vi "Pulse Fetch Data.vi"(0 "RFmx Session in":refnum<k21>, 11 "error in":errorcluster) -> (3 "Per Pulse Results (Header Name)":string[](array[string]), 4 "RFmx Session Out":refnum<k21>, 6 "Per Pulse Results (for MP)":dbl[][](array[numeric])=[[-60.19434452056885, -48.23559761047363, -61.500163078308105, -61.676697731018066, -50.09932041168213, -61.2670373916626, -47.940940856933594, -60.594682693481445, -54.222588539123535, -68.17487716674805], [-51.47902011871338, -63.676371574401855, -49.32386875152588, -42.60602951049805, -41.78941249847412, -56.57611846923828, -67.04894065856934, -44.43309783935547, -53.89562129974365, -45.59821605682373], [-50.93127727508545, -48.11325550079346, -49.06841278076172, -42.55256652832031, -41.191606521606445, -55.30652046203613, -47.88793087005615, -44.32924270629883, -51.04572772979736, -45.574283599853516], [0.7774313706217917, 0.7743052754564207, 0.6733820768651879, 0.6972024148638998, 0.6739289285829677, 0.8012453172128895, 0.7789831746751243, 0.81331101938709, 0.6993593760935255, 0.7751122603266651], [-0.04818759954671978, -0.17045354969029822, -0.2937592841444876, -0.18006245433349588, -0.30206692305208827, -0.23840372056041464, -0.22733917807886903, -0.2726908323785403, -0.20409866605988866, -0.22706977878895118], [1.8971785430084185, 1.7078184861447125, 1.6125145446758244, 1.6429880662265446, 1.7003339064410368, 1.645767369340552, 1.8225724908268657, 1.500202053052531, 1.816586601520762, 1.7434164608706486], [9.902169056670972e-09, 1.0171003831640633e-08, 1.0087378671871648e-08, 1.0018839745468426e-08, 1.0021453073999283e-08, 9.937162678335199e-09, 1.0113660404718986e-08, 9.936247799288367e-09, 1.0029181489475149e-08, 1.0014254033422958e-08], [1.1747647026741224e-08, 0.00010001147191839247, 0.00020001407632828564, 0.0003000116995963527, 0.00040001415077715896, 0.0005000116894758734, 0.0006000140392077577, 0.000700011761394561, 0.0008000141195439436, 0.000900014054837663], [1.0266075038352937e-08, 1.0210194009332553e-08, 9.96602777140197e-09, 1.0195131948175912e-08, 1.0214687343427613e-08, 1.0248380139892106e-08, 1.003600972591812e-08, 1.0209683835273609e-08, 1.0208458229471944e-08, 1.0051256216333969e-08], [2.0016060941649103e-05, 0.00012001605265167608, 0.0002200186251165217, 0.0003200161244125173, 0.00042001858918951285, 0.0005200161200707459, 0.000620018587380489, 0.0007200160772447398, 0.0008200186061427676, 0.0009200186490169424], [1.9999915173664064e-05, 1.9999928162649538e-05, 1.9999979315091006e-05, 1.9999962883326592e-05, 1.9999940266618827e-05, 1.9999970715330443e-05, 1.9999948164994597e-05, 1.999989449659788e-05, 1.9999961878396942e-05, 2.0000044728873845e-05], [8.000006128542082e-05, 8.000009557087724e-05, 8.000003688745302e-05, 8.000002009960112e-05, 8.000005863752275e-05, 8.000001971001538e-05, 8.000010310677254e-05, 8.000006664992009e-05, 8.000000105017845e-05, nan], [19.999919881828227, 19.999923415962357, 19.999976074586076, 19.99996628673531, 19.99994048578986, 19.999972630258657, 19.999937910673005, 19.999902267256314, 19.99996929267048, nan], [9.999997645908488e-05, 0.00010000002373352679, 0.00010000001620254403, 9.999998298292771e-05, 9.999999890414157e-05, 9.999999042534582e-05, 0.00010000005127176714, 9.999996114651797e-05, 9.99999629285754e-05, nan]], 8 "TS Intrapulse Stability":dbl[][](array[numeric]), 10 "TS P2P Stability":dbl[][](array[numeric]), 14 "TS Acquired Amplitude":dbl[][](array[numeric]), 15 "error out":errorcluster)   [LabVIEW 2023]
uses:
  <vilib>/RFmx/Pulse/mx/RFmxPulse.llb/RFmxPulse Fetch Intrapulse Stability Trace.vi
  <vilib>/RFmx/Pulse/mx/RFmxPulse.llb/RFmxPulse Fetch Pulse To Pulse Stability Trace.vi
  <vilib>/RFmx/Pulse/mx/RFmxPulse.llb/RFmxPulse Fetch Acquired Amplitude Trace.vi
  <resource>/objmgr/RFmxPulse.rc
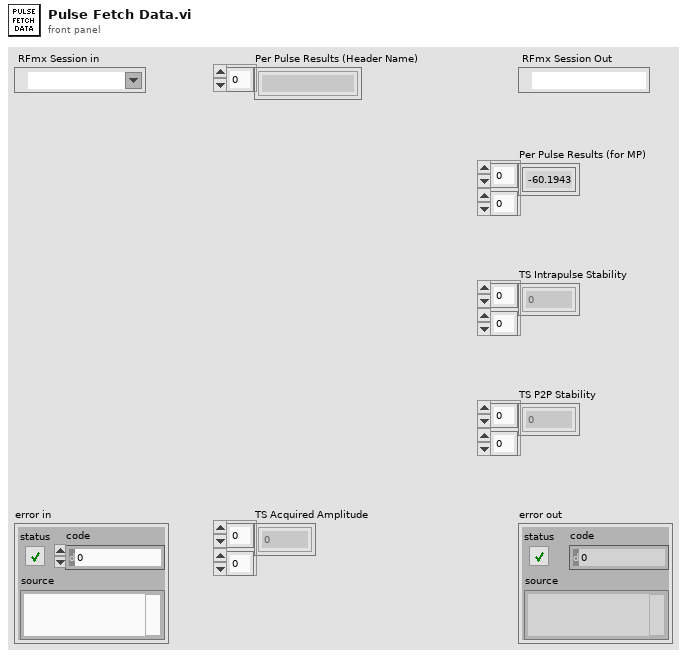
[diagram p1: front panel]
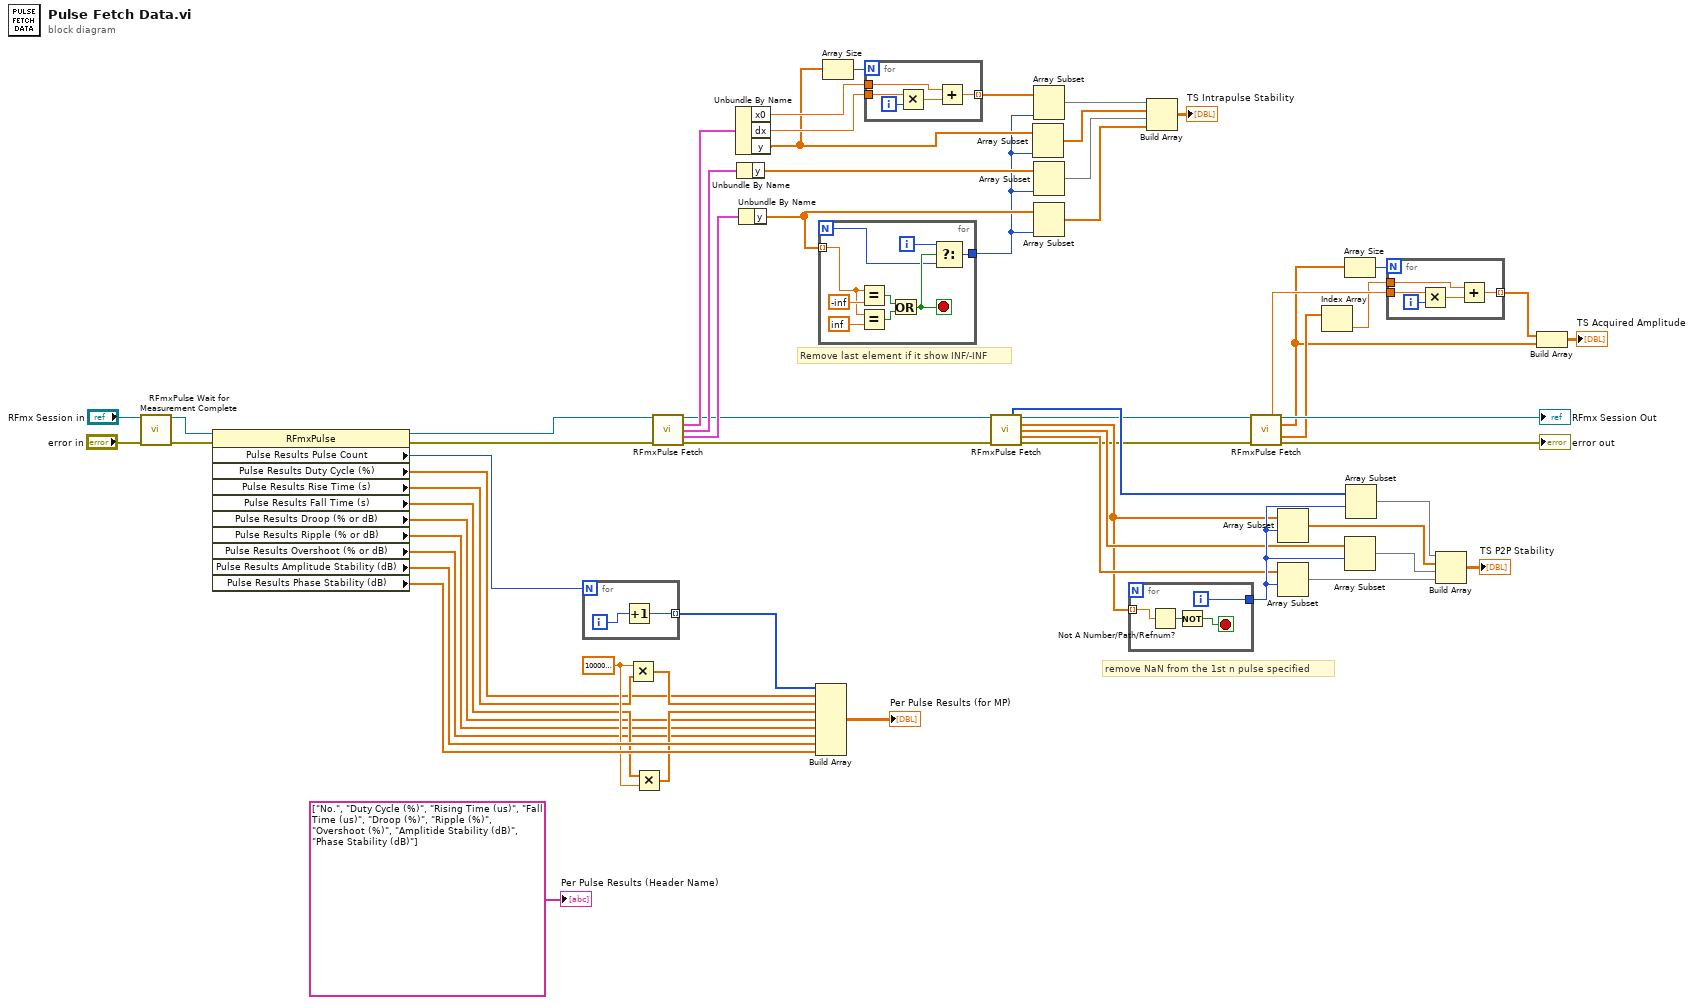
[diagram p0: block diagram]
diagram:
  w30 = 1000000.0
  # "Remove last element if it show INF/-INF"
  # "remove NaN from the 1st n pulse specified"
  n1 = call <vilib>:"RFmxPulse Wait for Measurement Complete.vi"("Instrument Handle In"="RFmx Session in", "error in (no error)"="error in") -> ("Instrument Handle Out"=w17:refnum<k21>, "error out"=w16:errorcluster)  [unwired: 12 in]
  n2 = property class="RFmxPulse"(reference=w17, error in=w16) -> (reference out=w13:refnum<k21>, error out=w14:errorcluster, "Pulse Results Pulse Count"=w37:i32, "Pulse Results Duty Cycle (%)"=w21:dbl[], "Pulse Results Rise Time (s)"=w26:dbl[], "Pulse Results Fall Time (s)"=w28:dbl[], "Pulse Results Droop (% or dB)"=w22:dbl[], "Pulse Results Ripple (% or dB)"=w23:dbl[], "Pulse Results Overshoot (% or dB)"=w24:dbl[], "Pulse Results Amplitude Stability (dB)"=w39:dbl[], "Pulse Results Phase Stability (dB)"=w40:dbl[])
  n3 = for {
    N: w37 -> [_]
    tunnel: [w61] -> w38 mode=indexing
    i -> [w62]
    n4 = Increment(x=w62) -> (x+1=w61:i32)
  }
  n5 = Multiply(x=w30, y=w26) -> (x*y=w27:dbl[])
  n6 = Multiply(x=w28, y=w30) -> (x*y=w29:dbl[])
  n7 = call-poly <vilib>:"RFmxPulse Fetch.vi"("Instrument Handle In"=w13, "error in (no error)"=w14) -> ("Instrument Handle Out"=w18:refnum<k21>, "Intrapulse Amplitude Stability (dB)"=w49:cluster{"x0":dbl, "dx":dbl, "y":sgl[]}, "Intrapulse Phase Stability (dB)"=w47:cluster{"x0":dbl, "dx":dbl, "y":sgl[]}, "Intrapulse Total Stability (dB)"=w45:cluster{"x0":dbl, "dx":dbl, "y":sgl[]}, "error out"=w19:errorcluster)  [unwired: 9 in]
  n8 = Unbundle By Name(w49) -> ("x0"=w53:dbl, "dx"=w52:dbl, "y"=w51:sgl[])
  n9 = Unbundle By Name(w47) -> ("y"=w48:sgl[])
  n10 = Unbundle By Name(w45) -> ("y"=w46:sgl[])
  n11 = Build Array(w38, w21, w27, w29, w22, w23, w24, w39, w40) -> (→"Per Pulse Results (for MP)":dbl[][])
  n12 = for {
    N -> [w63]
    tunnel: w46 -> [w70] mode=indexing
    tunnel: [w65] -> w36
    i -> [w64]
    stop <- w66 stop-if-true
    n13 = Equal?(x=w70, y=-inf) -> (x = y?=w68:bool)
    n14 = Equal?(x=w70, y=inf) -> (x = y?=w67:bool)
    n15 = Or(x=w68, y=w67) -> (x .or. y?=w66:bool)
    n16 = Select(t=w64, s=w66, f=w63) -> (s? t:f=w65:i32)
  }
  n17 = Array Size(array=w51) -> (size(s)=w50:i32)
  n18 = for {
    N: w50 -> [_]
    tunnel: w52 -> [w76]
    tunnel: w53 -> [w73]
    tunnel: [w72] -> w54 mode=indexing
    i -> [w75]
    n19 = Multiply(x=w76, y=w75) -> (x*y=w74:dbl)
    n20 = Add(x=w73, y=w74) -> (x+y=w72:dbl)
  }
  n21 = call-poly <vilib>:"RFmxPulse Fetch.vi"("Instrument Handle In"=w18, "error in (no error)"=w19) -> ("Pulse Index"=w31:i32[], "Instrument Handle Out"=w11:refnum<k21>, "Pulse To Pulse Amplitude Stability (dB)"=w32:dbl[], "Pulse To Pulse Phase Stability (dB)"=w33:dbl[], "Pulse To Pulse Total Stability (dB)"=w34:dbl[], "error out"=w10:errorcluster)  [unwired: 8 in]
  n22 = Array Subset(array=w51, length=w36) -> (w42:sgl[])  [unwired: 1 in]
  n23 = Array Subset(array=w54, length=w36) -> (w41:dbl[])  [unwired: 1 in]
  n24 = Array Subset(array=w48, length=w36) -> (w43:sgl[])  [unwired: 1 in]
  n25 = Array Subset(array=w46, length=w36) -> (w44:sgl[])  [unwired: 1 in]
  n26 = for {
    tunnel: w32 -> [w80] mode=indexing
    tunnel: [w77] -> w35
    i -> [w77]
    stop <- w78 stop-if-true
    n27 = Not A Number/Path/Refnum?(number/path/refnum=w80) -> (NaN/Path/Refnum?=w79:bool)
    n28 = Not(x=w79) -> (.not. x?=w78:bool)
  }
  n29 = Build Array(w41, w42, w43, w44) -> (→"TS Intrapulse Stability":dbl[][])
  n30 = call-poly <vilib>:"RFmxPulse Fetch.vi"("Instrument Handle In"=w11, "error in (no error)"=w10) -> ("Sample Duration (s)"=w6:dbl, "Instrument Handle Out"=→"RFmx Session Out":refnum<k21>, "Amplitude"=w2:sgl[], "Start Time Stamp (s)"=w5:dbl[], "error out"=→"error out":errorcluster)  [unwired: 8 in, 1 out]
  n31 = Array Subset(array=w32, index=w35) -> (w57:dbl[])  [unwired: 1 in]
  n32 = Array Subset(array=w34, index=w35) -> (w59:dbl[])  [unwired: 1 in]
  n33 = Index Array(array=w5) -> (element=w4:dbl)  [unwired: 1 in]
  n34 = Array Size(array=w2) -> (size(s)=w7:i32)
  n35 = Array Subset(array=w33, index=w35) -> (w58:dbl[])  [unwired: 1 in]
  n36 = Array Subset(array=w31, index=w35) -> (w56:i32[])  [unwired: 1 in]
  n37 = for {
    N: w7 -> [_]
    tunnel: w6 -> [w85]
    tunnel: w4 -> [w82]
    tunnel: [w81] -> w3 mode=indexing
    i -> [w84]
    n38 = Multiply(x=w85, y=w84) -> (x*y=w83:dbl)
    n39 = Add(x=w82, y=w83) -> (x+y=w81:dbl)
  }
  n40 = Build Array(w56, w57, w58, w59) -> (→"TS P2P Stability":dbl[][])
  n41 = Build Array(w3, w2) -> (→"TS Acquired Amplitude":dbl[][])
  "Per Pulse Results (Header Name)" <- string[] ["No.", "Duty Cycle (%)", "Rising Time (us)", "Fall Time (us)", "Droop (%)", "Ripple (%)", "Overshoot (%)", "Amplitide Stability (dB)", "Phase Stability (dB)"]
